vi "XY to Waveform (single).vi"(8 "error in (no error)":errorcluster, 11 "XY-data in":cluster{"X-array":dbl[], "Y-array":dbl[]} {"Y-array" format="%.2p"; "X-array" format="%.2p"}) -> (0 "error out":errorcluster, 2 "Waveform cluster":cluster{"x0":dbl, "dx":dbl, "Y array":dbl[]}, 3 "Waveform out":waveform(dbl))   [LabVIEW 2019, in "xy_utilities.lvlib"]
doc: "Convert <b>XY-data</b> to <b>Waveform</b>."
uses:
  xy_utilities.lvlib
  Get X and Y (single).vi
  Resample (single).vi
  <vilib>/measure/maresamp.llb/Resample Waveforms (single shot).vi
  <vilib>/measure/maresamp.llb/Resample Pair of Arrays (single shot).vi
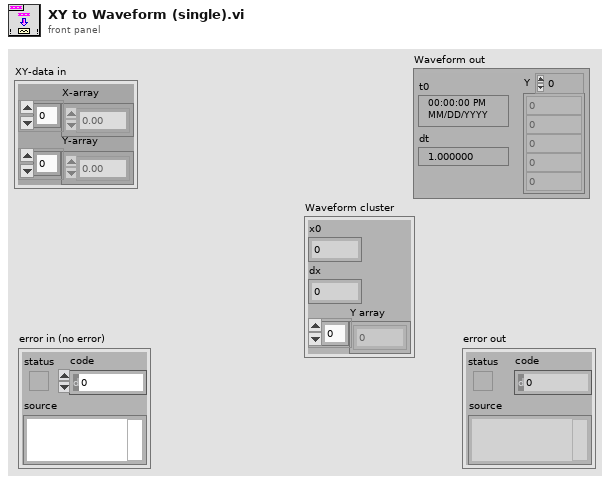
[diagram p1: front panel]
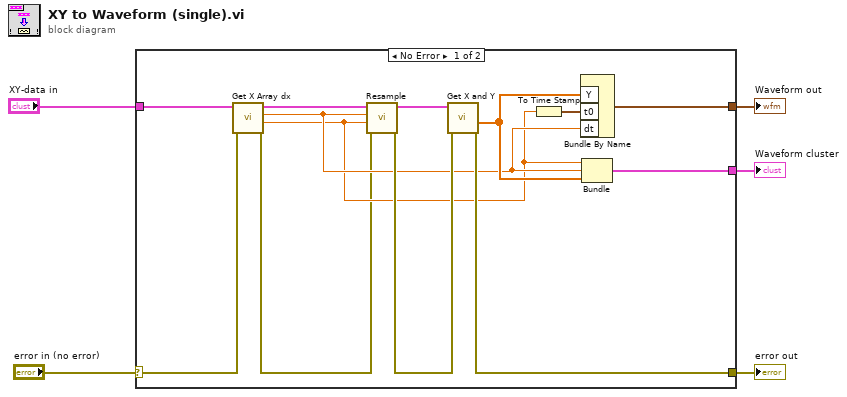
[diagram p0: block diagram]
diagram:
  n1 = case shown="No Error" "error in (no error)" {
    selector: "error in (no error)" -> [w7 w19]
    tunnel: [w18 w19] -> w4
    tunnel: "XY-data in" -> [w8 _]
    tunnel: [w15 _] -> w1
    tunnel: [w12 _] -> w2
    frame No Error {
      n2 = call "Get X Array dx.vi"("error in (no error)"=w7, "XY-data"=w8) -> ("error out"=w6:errorcluster, "X0"=w10:dbl, "dX"=w11:dbl, "XY-data out"=w9:cluster{"X-array":dbl[], "Y-array":dbl[]})  [unwired: 6 in]
      n3 = call-poly "Resample.vi"("error in (no error)"=w6, "t0"=w10, "dt"=w11, "XY-data"=w9) -> ("error out"=w16:errorcluster, "Resampled XY-data out"=w17:cluster{"X-array":dbl[], "Y-array":dbl[]})  [unwired: 6 in]
      n4 = call-poly "Get X and Y.vi"("error in (no error)"=w16, "XY-data"=w17) -> ("error out"=w18:errorcluster, "Y-array"=w14:dbl[])  [unwired: 6 in, 2 out]
      n5 = To Time Stamp(1:w10) -> (0:w13:timestamp)
      n6 = Bundle By Name("Y"=w14, "t0"=w13, "dt"=w11) -> (w12:waveform(dbl))  [unwired: 1 in]
      n7 = Bundle("X0"=w10, "dX"=w11, "Y-array"=w14) -> (w15:cluster{"X0":dbl, "dX":dbl, "Y-array":dbl[]})  [unwired: 1 in]
    }
    frame Error {
    }
  }
  "error out" <- w4
  "Waveform out" <- w2
  "Waveform cluster" <- w1
